vi "update Segment.vi"(7 "Segment.lvclass":refnum<class "Segment.lvclass">, 8 "error in (no error)":errorcluster, 10 "Index":i32, 11 "Test in":refnum<class "Test.lvclass">) -> (0 "error out":errorcluster, 3 "Test out":refnum<class "Test.lvclass">)   [LabVIEW 2013]
uses:
  Test.lvclass
  Segment/Segment.lvclass
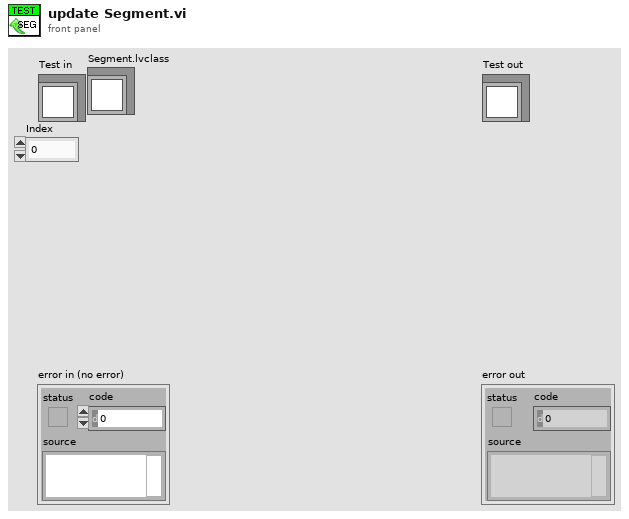
[diagram p1: front panel]
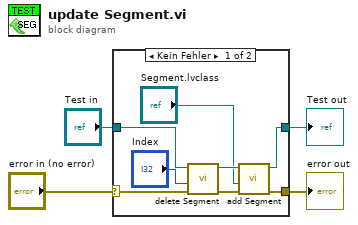
[diagram p0: block diagram]
diagram:
  n1 = case shown="Kein Fehler" "error in (no error)" {
    selector: "error in (no error)" -> [w11 w14]
    tunnel: [w5 w14] -> w3
    tunnel: [w6 w13] -> w1
    tunnel: "Test in" -> [w12 w13]
    frame No Error {
      n2 = call-dynamic "delete Segment.vi"("error in (no error)"=w11, "Index"="Index", "Test Eingang"=w12) -> ("error out"=w7:errorcluster, "Test Ausgang"=w9:refnum<class "Test.lvclass">)  [unwired: 7 in]
      n3 = call-dynamic "add Segment.vi"("error in (no error)"=w7, "Segment.lvclass"="Segment.lvclass", "Test Eingang"=w9) -> ("error out"=w5:errorcluster, "Test Ausgang"=w6:refnum<class "Test.lvclass">)  [unwired: 7 in]
    }
    frame Error {
    }
  }
  "error out" <- w3
  "Test out" <- w1
